vi "DAQ.Create Sample Clock.vi"(8 "error in (no error)":errorcluster, 11 "Instrument.DAQ":refnum<class "Instrument.DAQ.lvclass">) -> (0 "error out":errorcluster, 3 "Instrument.DAQ":refnum<class "Instrument.DAQ.lvclass">)   [LabVIEW 2019, in "Instrument.DAQ.lvclass"]
uses:
  Instrument.DAQ.lvclass
  Instrument.DAQ.lvclass/Instrument.DAQ.ctl
  <vilib>/DAQmx/configure/timing.llb/DAQmx Timing (Sample Clock).vi
  <resource>/objmgr/daqmx.rc
panel:
  out "Output.Onboard Buffer":u32[](array[numeric])
  out "Output.Buffer":u32[](array[numeric])
  out "Input.Onboard Buffer":u32[](array[numeric])
  out "Input.Buffer":u32[](array[numeric])
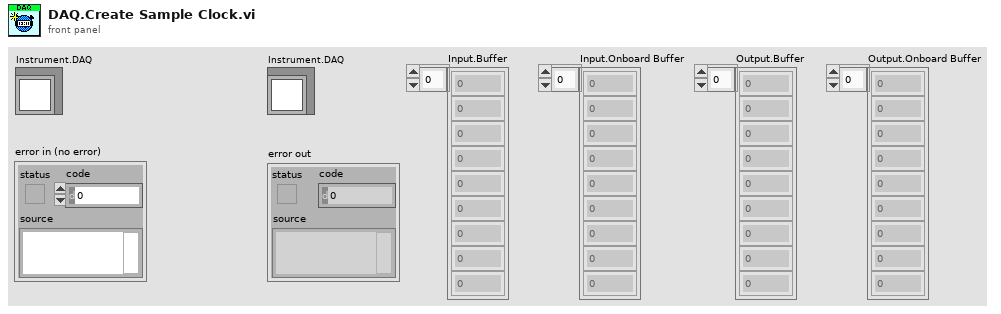
[diagram p1: front panel]
types:
  T1 = typedef "Instrument.DAQ.lvclass/DAQ.Sampling.Sample Mode--Ring.ctl" = i32
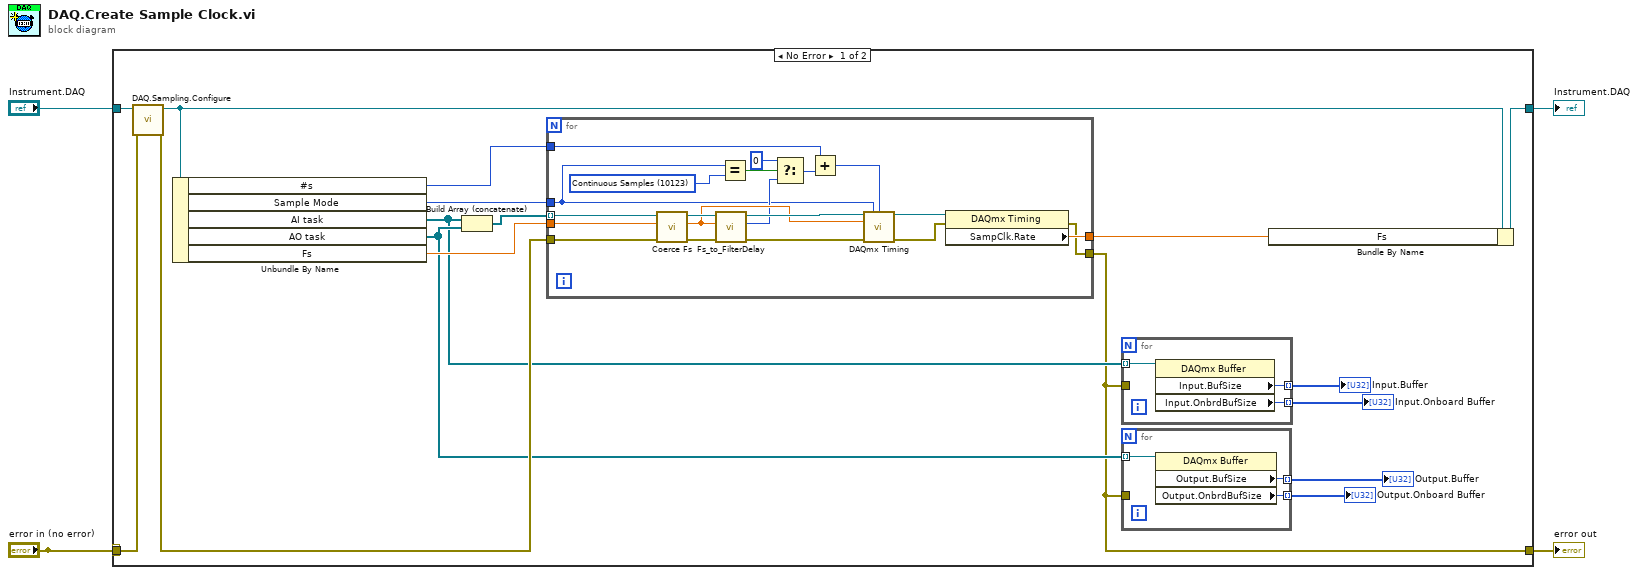
[diagram p0: block diagram]
diagram:
  n1 = case shown="No Error" "error in (no error)" {
    selector: "error in (no error)" -> [_ w49]
    tunnel: [w5 w49] -> w4
    tunnel: [w20 w48] -> w2
    tunnel: "Instrument.DAQ" -> [w16 w48]
    tunnel: "error in (no error)" -> [w17 _]
    frame No Error {
      n2 = call "DAQ.Sampling.Configure.vi"("error in (no error)"=w17, "Instrument.DAQ"=w16) -> ("error out"=w14:errorcluster, "Instrument.DAQ out"=w15:refnum<class "Instrument.DAQ.lvclass">)  [unwired: 8 in]
      n3 = Unbundle By Name(w15) -> ("#s"=w18:i32, "Sample Mode"=w19:T1, "AI task"=w6:refnum<k21>[], "AO task"=w11:refnum<k21>[], "Fs"=w13:dbl)
      n4 = Build Array (concatenate)(w6, w11) -> (w12:refnum<k21>[])
      n5 = for {
        tunnel: w12 -> [w41] mode=indexing
        tunnel: w13 -> [w37]
        tunnel: w14 -> [w38]
        tunnel: [w35] -> w5
        tunnel: [w39] -> w21
        tunnel: w19 -> [w22]
        tunnel: w18 -> [w26]
        w28 = 10123 items=["Finite Samples"=10178, "Continuous Samples"=10123] ("sample mode 2")
        n6 = call "Coerce Fs.vi"("error in (no error)"=w38, "Fs"=w37, "Refnum in"=w41) -> ("error out"=w32:errorcluster, "coerced(Fs)"=w30:dbl, "Refnum out"=w34:refnum<k21>)  [unwired: 6 in]
        n7 = call "Fs_to_FilterDelay.vi"("error in (no error)"=w32, "Fs"=w30, "Refnum in"=w34) -> ("error out"=w31:errorcluster, "Total Filter Delay (samples)"=w24:i32, "Refnum out"=w33:refnum<k21>)  [unwired: 6 in]
        n8 = Equal?(x=w22, y=w28) -> (x = y?=w29:bool)
        n9 = Select(t=0 ("f"), s=w29, f=w24) -> (s? t:f=w27:i32)
        n10 = Add(x=w26, y=w27) -> (x+y=w23:i32)
        n11 = call-poly <vilib>:"DAQmx Timing.vi"("task/channels in"=w33, "sample mode"=w22, "samples per channel"=w23, "rate"=w30, "error in"=w31) -> ("task out"=w40:refnum<k21>, "error out"=w36:errorcluster)  [unwired: 9 in]
        n12 = property class="DAQmx Timing"(reference=w40, error in=w36) -> (error out=w35:errorcluster, "SampClk.Rate"=w39:dbl)  [unwired: 1 out]
      }
      n13 = for {
        tunnel: w6 -> [w47] mode=indexing
        tunnel: [w46] -> w10 mode=indexing
        tunnel: [w45] -> w9 mode=indexing
        tunnel: w5 -> [_]
        n14 = property class="DAQmx Buffer"(reference=w47) -> ("Input.BufSize"=w46:u32, "Input.OnbrdBufSize"=w45:u32)  [unwired: 1 in, 2 out]
      }
      "Input.Buffer" <- w10
      "Input.Onboard Buffer" <- w9
      n15 = for {
        tunnel: w11 -> [w44] mode=indexing
        tunnel: [w43] -> w8 mode=indexing
        tunnel: [w42] -> w7 mode=indexing
        tunnel: w5 -> [_]
        n16 = property class="DAQmx Buffer"(reference=w44) -> ("Output.BufSize"=w43:u32, "Output.OnbrdBufSize"=w42:u32)  [unwired: 1 in, 2 out]
      }
      "Output.Buffer" <- w8
      "Output.Onboard Buffer" <- w7
      n17 = Bundle By Name(cluster=w15, "Fs"=w21) -> (w20:refnum<class "Instrument.DAQ.lvclass">)
    }
    frame Error {
    }
  }
  "error out" <- w4
  "Instrument.DAQ" <- w2
